vi "Rotate Rectangle.vi"(8 "Angle":dbl, 10 "Rectangle":cluster{dbl, dbl, dbl, dbl}) -> (2 "polygon":cluster{dbl, dbl}[](array[cluster]))   [LabVIEW 2019]
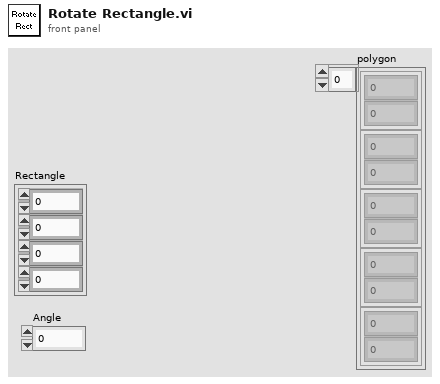
[diagram p1: front panel]
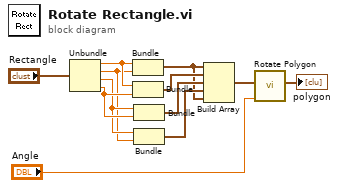
[diagram p0: block diagram]
diagram:
  n1 = Unbundle("Rectangle") -> (w6:dbl, w4:dbl, w5:dbl, w11:dbl)
  n2 = Bundle(w6, w4) -> (w7:cluster{dbl, dbl})  [unwired: 1 in]
  n3 = Bundle(w6, w11) -> (w10:cluster{dbl, dbl})  [unwired: 1 in]
  n4 = Bundle(w5, w11) -> (w9:cluster{dbl, dbl})  [unwired: 1 in]
  n5 = Bundle(w5, w4) -> (w8:cluster{dbl, dbl})  [unwired: 1 in]
  n6 = Build Array(w7, w10, w9, w8, w7) -> (w3:cluster{dbl, dbl}[])
  n7 = call "Rotate Polygon.vi"("Angle"="Angle", "polygon 2"=w3) -> ("polygon"=→"polygon":cluster{dbl, dbl}[])  [unwired: 9 in]
